vi "ziImpedanceCalibObtain.vi"(6 "Ref_Z":cdb[](array[numeric]), 7 "Ref ID":i16(ring)=1 items=["Open"=-2, "Short"=-1, "R"=1, "C"=2, "L"=3, "R || C"=4], 8 "Measurement (F,Z0,..,Zn)":dbl[][](array[numeric]) format="%#_6p") -> (3 "ziCalib":T1)   [LabVIEW 2009, in "Zurich Instruments LabOne.lvlib"]
doc: "Obtain calibration data from a reference measurement."
uses:
  <instrlib>/Zurich Instruments LabOne/Zurich Instruments LabOne.lvlib
  <instrlib>/Zurich Instruments LabOne/Public/Utility/Impedance/ziTypeCalib.ctl
  <instrlib>/Zurich Instruments LabOne/Public/Utility/Impedance/ziTypeCalibModel.ctl
panel:
  out "Calibration Theta (deg)":T3(graph)
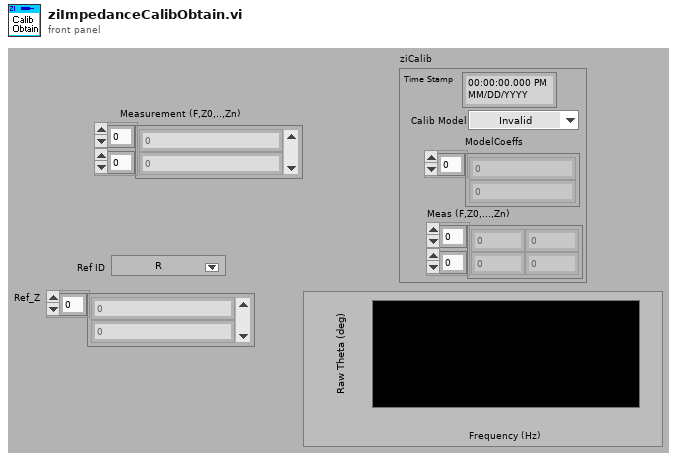
[diagram p1: front panel]
types:
  T1 = typedef "Zurich Instruments LabOne.lvlib/ziTypeCalib.ctl" = cluster{"Time Stamp":timestamp, "Calib Model":T2, "ModelCoeffs":cdb[], "Meas (F,Z0,...,Zn)":dbl[][]}
  T2 = typedef "Zurich Instruments LabOne.lvlib/ziTypeCalibModel.ctl" = enum16{"Invalid", "Unity", "R||C", "R||L", "R*C", "R*L"}
  T3 = cluster{"Output (F,X1,Y1,X2,Y2,...,Vo)":dbl[], dbl[]}
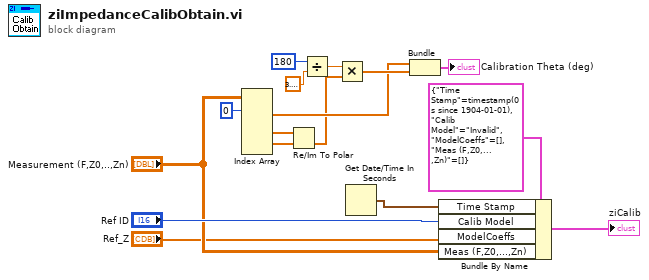
[diagram p0: block diagram]
diagram:
  n1 = Index Array(array="Measurement (F,Z0,..,Zn)", index (row) #1=0 ("index (row)")) -> (element #1=w10:dbl[], element #2=w9:dbl[], element #3=w8:dbl[])  [unwired: 5 in]
  n2 = Re/Im To Polar(2:w8, 3:w9) -> (0:w7:dbl[])  [unwired: 1 out]
  n3 = Divide(x=180, y=3.141592653589793) -> (x/y=w13:dbl)
  n4 = Multiply(x=w13, y=w7) -> (x*y=w15:dbl[])
  n5 = Get Date/Time In Seconds() -> (seconds since 1Jan1904=w1:timestamp)
  n6 = Bundle("Measurement (F,Z0,..,Zn)"=w10, w15) -> (→"Calibration Theta (deg)":cluster{"Measurement (F,Z0,..,Zn)":dbl[], dbl[]})  [unwired: 1 out]
  n7 = Bundle By Name(cluster=T1 {"Time Stamp"=timestamp(0 s since 1904-01-01), "Calib Model"=enum."Invalid", "ModelCoeffs"=[], "Meas (F,Z0,...,Zn)"=[]} ("ziCalib"), "Time Stamp"=w1, "Calib Model"="Ref ID", "ModelCoeffs"="Ref_Z", "Meas (F,Z0,...,Zn)"="Measurement (F,Z0,..,Zn)") -> (→"ziCalib":T1)
